vi "4.3.vi"() -> ()   [LabVIEW 2017]
panel:
  out "平方根":dbl
  in  "输入值":dbl
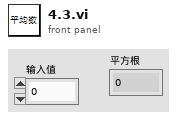
[diagram p1: front panel]
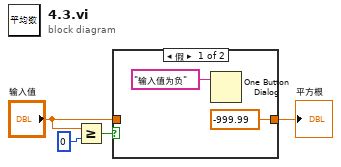
[diagram p0: block diagram]
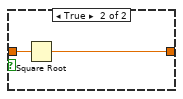
[diagram p2: hidden frame]
diagram:
  n1 = Greater Or Equal?(x="输入值", y=0) -> (x >= y?=w2:bool)
  n2 = case shown="假" w2 {
    tunnel: "输入值" -> [_ w8]
    tunnel: [-999.99 w7] -> w1
    frame False {
      n3 = One Button Dialog(message="输入值为负" ("消息")) -> ()  [unwired: 1 in, 1 out]
    }
    frame True {
      n4 = Square Root(x=w8) -> (sqrt(x)=w7:dbl)
    }
  }
  "平方根" <- w1
